vi "Get Service Interface.vi"(8 "error in (no error)":errorcluster, 11 "MeasurementServiceV1 in":refnum<class "Measurement Service V1.lvclass">) -> (0 "error out":errorcluster, 2 "service interface":string, 3 "MeasurementServiceV1 out":refnum<class "Measurement Service V1.lvclass">)   [LabVIEW 2020, in "MeasurementLink Measurement Server.lvlib" / "Measurement Service V1.lvclass"]
uses:
  Measurement Service V1.lvclass
  Measurement Service V1.lvclass/Measurement Service V1.ctl
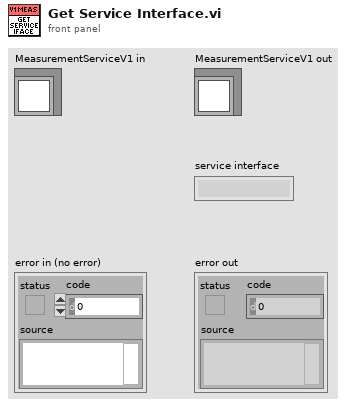
[diagram p1: front panel]
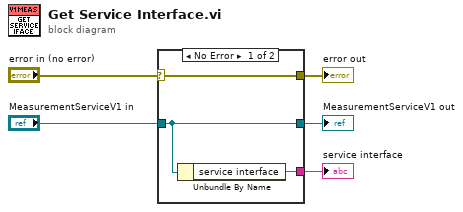
[diagram p0: block diagram]
diagram:
  n1 = case shown="No Error" "error in (no error)" {
    selector: "error in (no error)" -> [w8 w10]
    tunnel: [w8 w10] -> w4
    tunnel: [w7 w9] -> w2
    tunnel: "MeasurementServiceV1 in" -> [w7 w9]
    tunnel: [w6 _] -> w1
    frame No Error {
      n2 = Unbundle By Name(w7) -> ("service interface"=w6:string)
    }
    frame Error {
    }
  }
  "error out" <- w4
  "MeasurementServiceV1 out" <- w2
  "service interface" <- w1
